vi "Passing Paramters Complex Struct Corrected.vi"(8 "error in (no error)":errorcluster) -> (0 "error out":errorcluster, 3 "function return":i32)   [LabVIEW 2009, in "LabVIEWWrapper_PassingDataSampleDLL.lvlib"]
doc: "int PassingParamters_ComplexStruct (struct complexStructPolygon triangle);"
uses:
  LabVIEWWrapper_PassingDataSampleDLL.lvlib
  CustomControlsForStructs/ComplexStruct Polygon.ctl
  PassingDataSampleDLL.dll
panel:
  in  "ComplexStruct Polygon":T1={"name"="Triange", "numVertices"=3, "Vertices"=[{"x"=1, "y"=2}, {"x"=2, "y"=6}, {"x"=3, "y"=3}]}
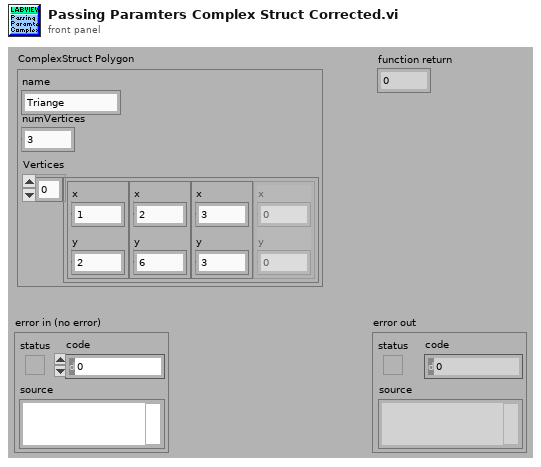
[diagram p1: front panel]
types:
  T1 = typedef "LabVIEWWrapper_PassingDataSampleDLL.lvlib/ComplexStruct Polygon.ctl" = cluster{"name":string, "numVertices":i32, "Vertices":cluster{"x":i32, "y":i32}[]}
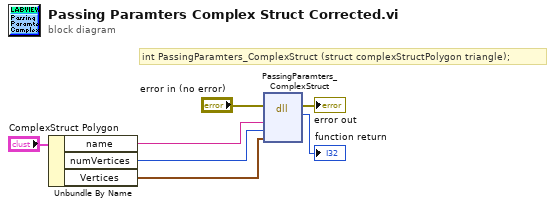
[diagram p0: block diagram]
diagram:
  # "int PassingParamters_ComplexStruct (struct complexStructPolygon triangle);"
  n1 = Unbundle By Name("ComplexStruct Polygon") -> ("name"=w3:string, "numVertices"=w2:i32, "Vertices"=w1:cluster{"x":i32, "y":i32}[])
  n2 = dll-call lib="C:/My Dropbox/Systems Engineering Application/SDK/C Integration/LabVIEWWrapper/PassingDataSampleDLL.*" fn="PassingParamters_ComplexStruct"(error in="error in (no error)", "name"=w3, "numVertices"=w2, "Vertices"=w1) -> (error out=→"error out":errorcluster, "return type"=→"function return":i32)  [unwired: 5 in, 1 out]
